vi "Log_Shutter.vi"(6 "command":string, 7 "domeState":string, 8 "pathLogDomeFile":string) -> ()   [LabVIEW 2018]
panel:
  out "Date":string
  in  "pathLogDomeFile":path
  out "error out":errorcluster
  out "writingLog":bool
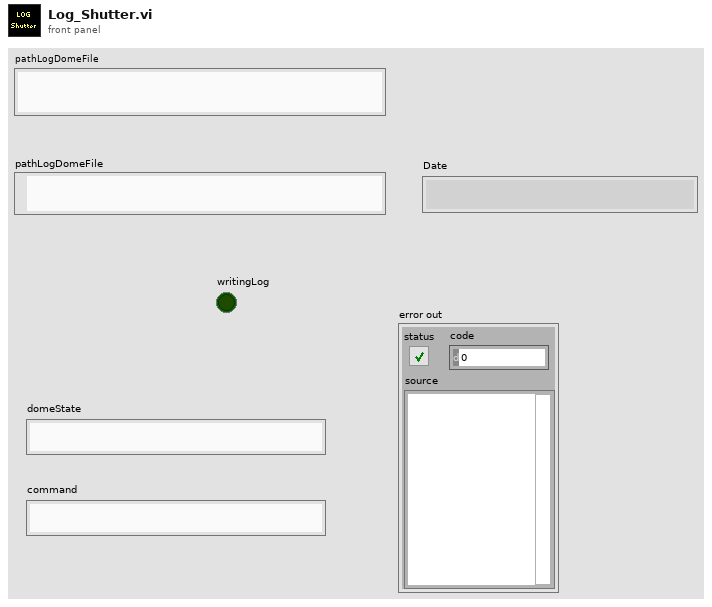
[diagram p1: front panel]
types:
  T1 = enum16{"open", "replace", "create", "open or create", "replace or create", "replace or create with confirmation"}
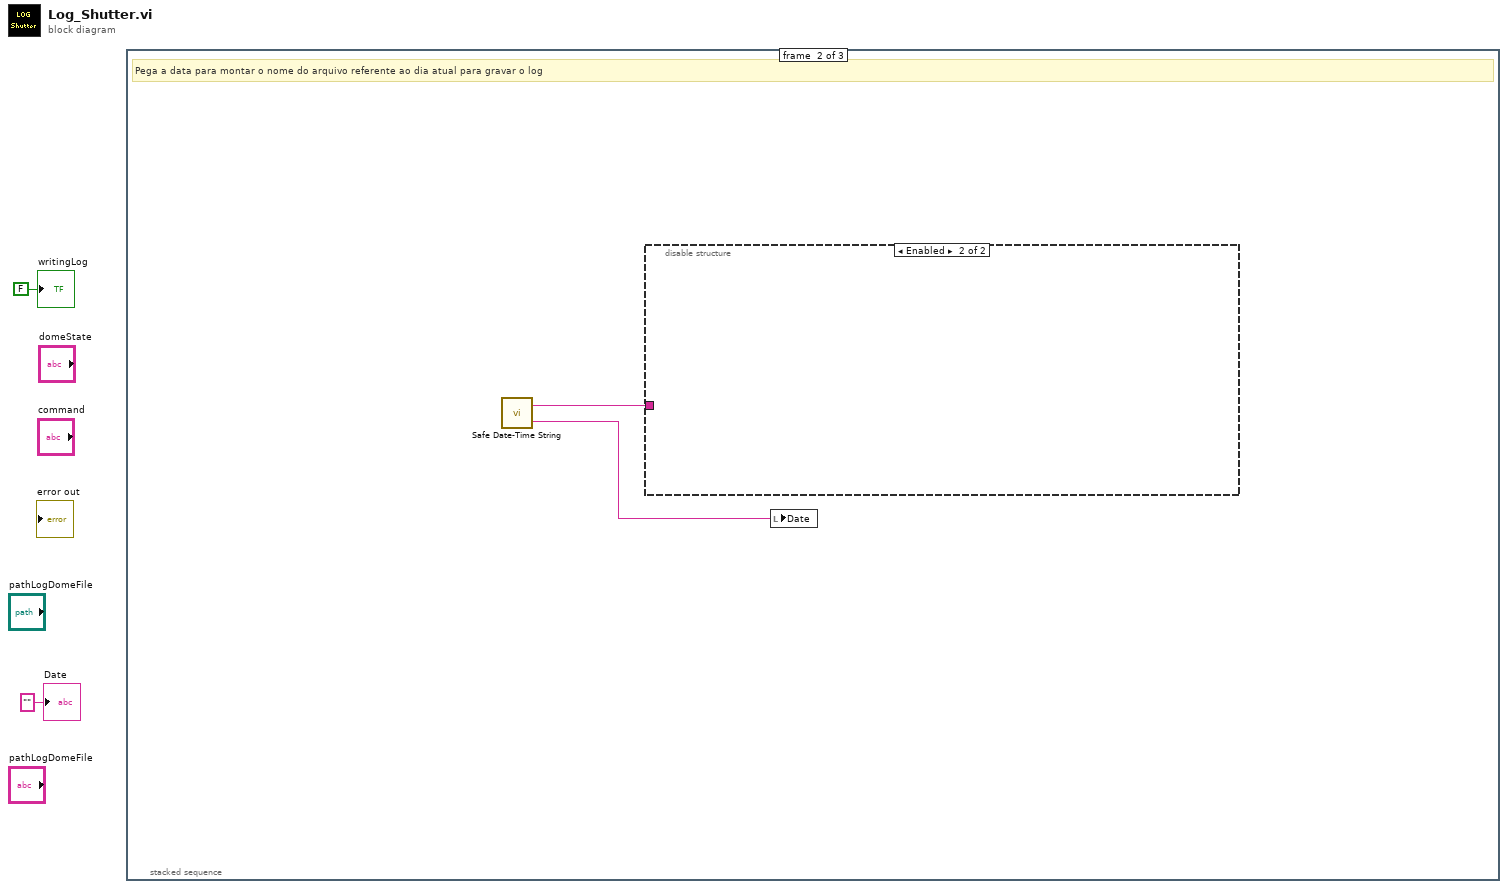
[diagram p0: block diagram]
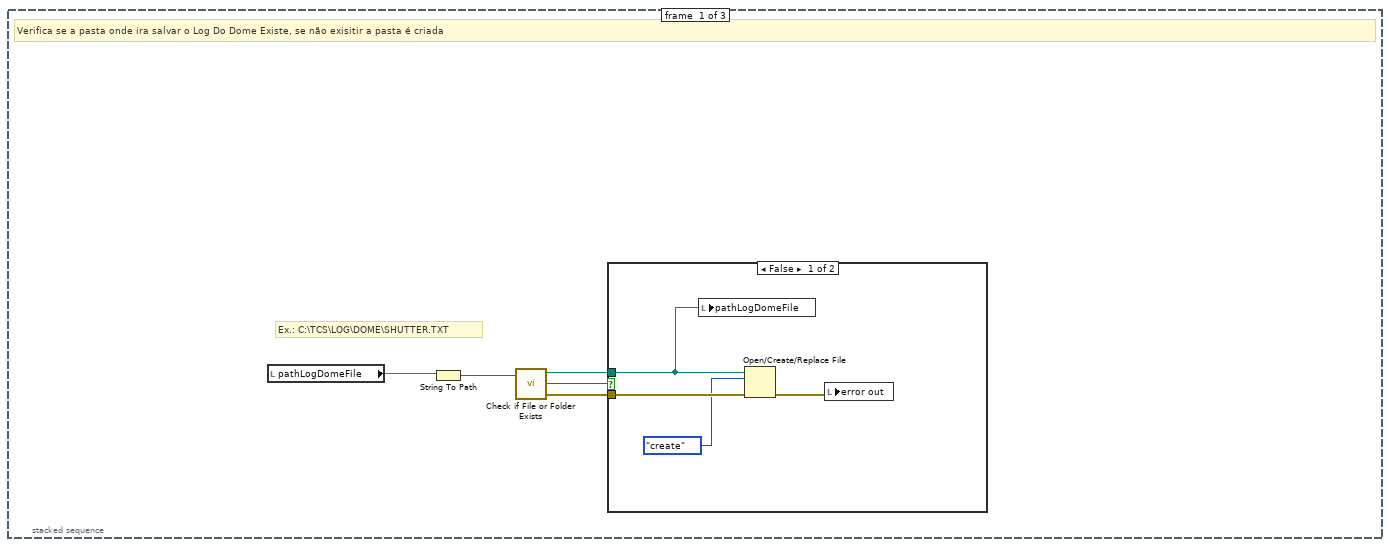
[diagram p2: hidden frame]
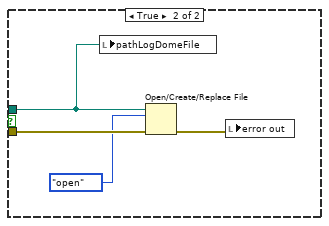
[diagram p3: hidden frame]
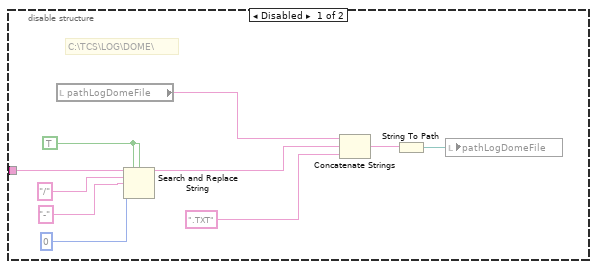
[diagram p4: hidden frame]
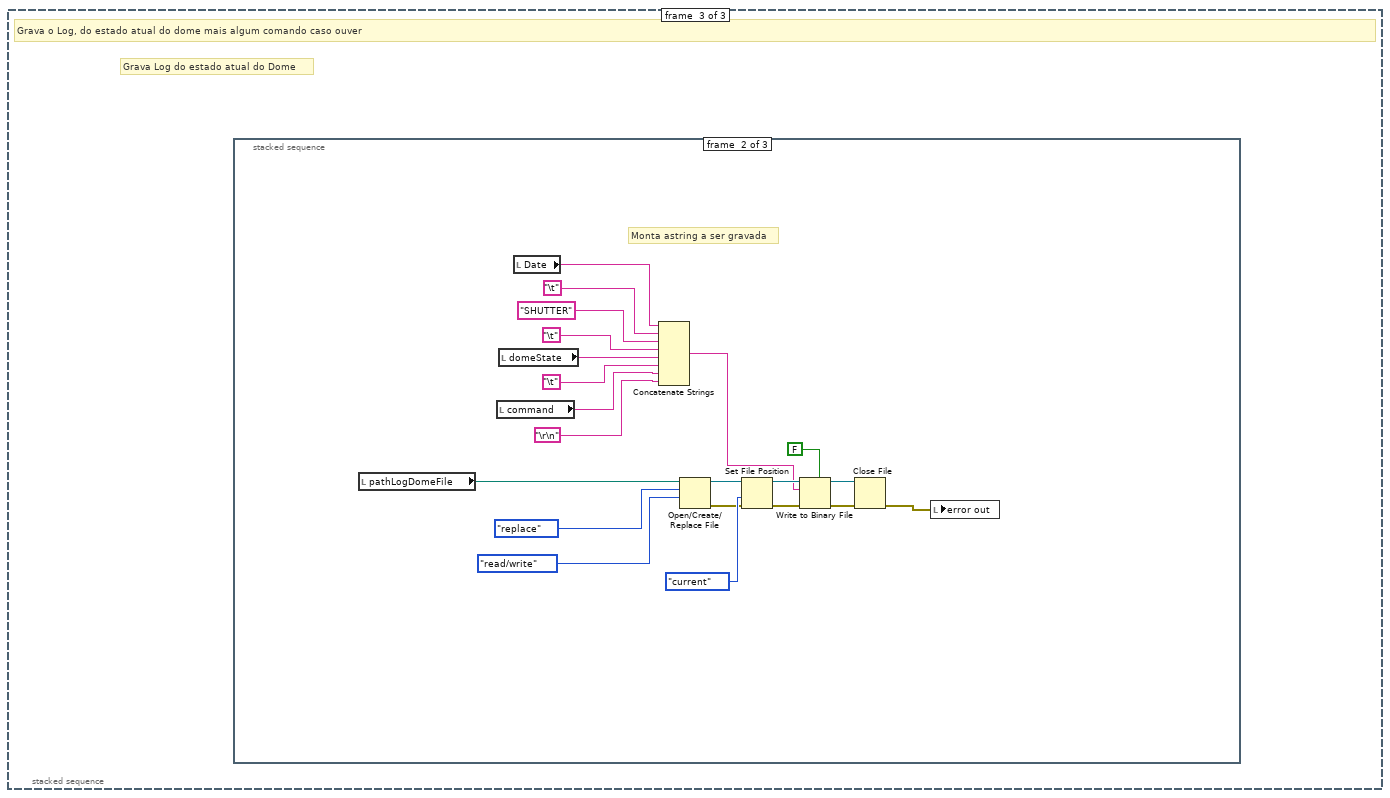
[diagram p5: hidden frame]
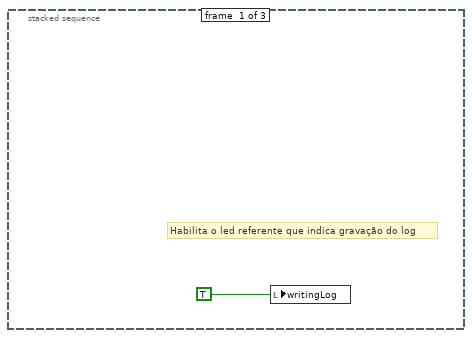
[diagram p6: hidden frame]
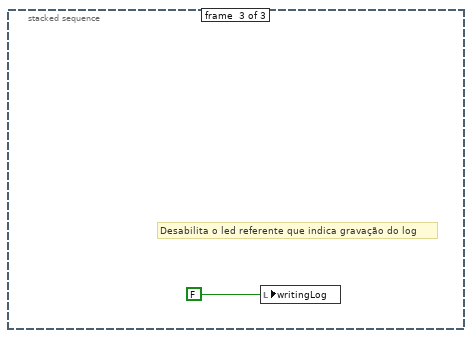
[diagram p7: hidden frame]
diagram:
  n1 = stacked-sequence {
    frame #0 {
      # "Ex.: C:\\TCS\\LOG\\DOME\\SHUTTER.TXT"
      # "Verifica se a pasta onde ira salvar o Log Do Dome Existe, se não exisitir a pasta é criada"
      n2 = local read "pathLogDomeFile"() -> (w4:string)
      n3 = String To Path(string=w4) -> (path=w3:path)
      n4 = call <vilib>:"Check if File or Folder Exists.vi"("path"=w3) -> ("error out"=w5:errorcluster, "file or folder exists?"=w7:bool, "dup path"=w6:path)  [unwired: 8 in]
      n5 = case shown="False" w7 {
        tunnel: w6 -> [w8 w12]
        tunnel: w5 -> [w11 w15]
        frame False {
          n6 = local write "pathLogDomeFile"(w8) -> ()
          n7 = Open/Create/Replace File(file path (use dialog)=w8, error in=w11, operation (0:open)=T1."create") -> (error out=w10:errorcluster)  [unwired: 3 in, 2 out]
          n8 = local write "error out"(w10) -> ()
        }
        frame True {
          n9 = local write "pathLogDomeFile"(w12) -> ()
          n10 = Open/Create/Replace File(file path (use dialog)=w12, error in=w15, operation (0:open)=T1."open") -> (error out=w14:errorcluster)  [unwired: 3 in, 2 out]
          n11 = local write "error out"(w14) -> ()
        }
      }
    }
    frame #1 {
      # "Pega a data para montar o nome do arquivo referente ao dia atual para gravar o log"
      n12 = call "Safe Date-Time String.vi"() -> ("Safe time string"=w17:string, "Safe date string"=w16:string)  [unwired: 3 in]
      n13 = disable-structure shown="Enabled" {
        disable-tunnel: w16 -> [w25 _]
        frame Disabled {
          w21 = TRUE ("replace all? (F)")
          # "C:\\TCS\\LOG\\DOME\\"
          n14 = local read "pathLogDomeFile"() -> (w18:string)
          n15 = Search and Replace String(replace all?=w21, case sensitive?=w21, input string=w25, search string="/" ("replace string (\"\")"), replace string="-" ("replace string (\"\")"), offset=0 ("offset (0)")) -> (result string=w19:string)  [unwired: 2 in, 3 out]
          n16 = Concatenate Strings(w18, w19, ".TXT" ("SOMENTE DIRETORIO")) -> (w26:string)
          n17 = String To Path(string=w26) -> (path=w20:path)
          n18 = local write "pathLogDomeFile"(w20) -> ()
        }
        frame Enabled {
        }
      }
      n19 = local write "Date"(w17) -> ()
    }
    frame #2 {
      # "Grava Log do estado atual do Dome"
      # "Grava o Log, do estado atual do dome mais algum comando caso ouver"
      n20 = stacked-sequence {
        frame #0 {
          # "Habilita o led referente que indica gravação do log"
          n21 = local write "writingLog"(TRUE) -> ()
        }
        frame #1 {
          # "Monta astring a ser gravada"
          n22 = local read "pathLogDomeFile"() -> (w49:path)
          n23 = local read "command"() -> (w31:string)
          n24 = local read "domeState"() -> (w38:string)
          n25 = local read "Date"() -> (w34:string)
          n26 = Concatenate Strings(w34, "\t", "SHUTTER", "\t", w38, "\t", w31, "\r\n") -> (w37:string)
          n27 = Open/Create/Replace File(file path (use dialog)=w49, operation (0:open)=T1."replace", access (0:read/write)=enum16{"read/write", "read-only", "write-only"}."read/write") -> (refnum out=w47:refnum<file>, error out=w43:errorcluster)  [unwired: 3 in, 1 out]
          n28 = Set File Position(refnum=w47, from (0:start)=enum16{"start", "end", "current"}."current", error in=w43) -> (refnum out=w44:refnum<file>, error out=w45:errorcluster)  [unwired: 1 in]
          n29 = Write to Binary File(file (use dialog)=w44, data=w37, error in=w45, 5:FALSE ("prepend array or string size? (T)")) -> (refnum out=w41:refnum<file>, error out=w40:errorcluster)  [unwired: 2 in, 1 out]
          n30 = Close File(refnum=w41, error in=w40) -> (error out=w39:errorcluster)  [unwired: 1 out]
          n31 = local write "error out"(w39) -> ()
        }
        frame #2 {
          # "Desabilita o led referente que indica gravação do log"
          n32 = local write "writingLog"(FALSE) -> ()
        }
      }
    }
  }
  "writingLog" <- FALSE ("writingLog")
  "Date" <- "" ("Date")
